vi "Default_Wash.vi"(0 "UI_Cluster_In":T1, 3 "error in":errorcluster) -> (7 "UI_Cluster_Out":T1, 10 "error out":errorcluster)   [LabVIEW 2020]
uses:
  controls/UI_Ref_Cluster.ctl
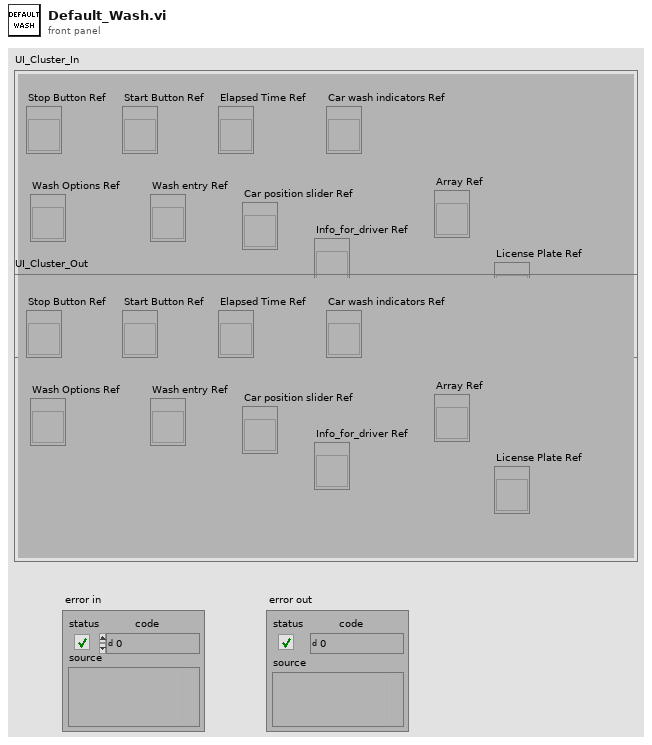
[diagram p1: front panel]
types:
  T1 = typedef "UI_Ref_Cluster.ctl" = cluster{"Stop Button Ref":refnum<vi>, "Start Button Ref":refnum<vi>, "Elapsed Time Ref":refnum<vi>, "Car wash indicators Ref":refnum<vi>, "Wash Options Ref":refnum<vi>, "Wash entry Ref":refnum<vi>, "Car position slider Ref":refnum<vi>, "Info_for_driver Ref":refnum<vi>, "Array Ref":refnum<vi>, "License Plate Ref":refnum<vi>}
  T2 = enum8{"Enabled", "Disabled", "Disabled and Grayed Out"}
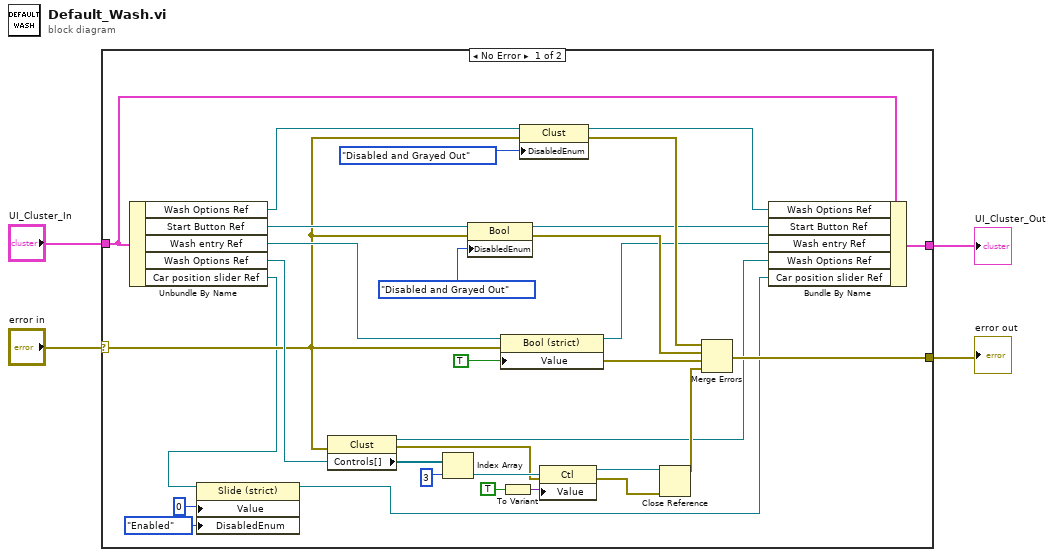
[diagram p0: block diagram]
diagram:
  n1 = case shown="No Error" "error in" {
    selector: "error in" -> [w15 w37]
    tunnel: [w21 w37] -> w3
    tunnel: "UI_Cluster_In" -> [w35 w36]
    tunnel: [w34 w36] -> w1
    frame No Error {
      n2 = Unbundle By Name(w35) -> ("Wash Options Ref"=w30:refnum<vi>, "Start Button Ref"=w27:refnum<vi>, "Wash entry Ref"=w24:refnum<vi>, "Wash Options Ref"=w20:refnum<vi>, "Car position slider Ref"=w7:refnum<vi>)
      n3 = property class="Slide (strict)"(reference=w7, "Value"=i8 0, "DisabledEnum"=T2."Enabled" ("Disabled")) -> (reference out=w6:refnum<vi>)  [unwired: 1 in, 1 out]
      n4 = property class="Clust"(reference=w20, error in=w15) -> (reference out=w9:refnum<vi>, error out=w14:errorcluster, "Controls[]"=w13:refnum<vi>[])
      n5 = Index Array(array=w13, index=3) -> (element=w18:refnum<vi>)
      n6 = property class="Bool"(reference=w27, error in=w15, "DisabledEnum"=T2."Disabled and Grayed Out" ("Disabled")) -> (reference out=w26:refnum<vi>, error out=w25:errorcluster)
      n7 = property class="Bool (strict)"(reference=w24, error in=w15, "Value"=TRUE) -> (reference out=w23:refnum<vi>, error out=w22:errorcluster)
      n8 = To Variant(anything=TRUE) -> (Variant=w16:variant)
      n9 = property class="Clust"(reference=w30, error in=w15, "DisabledEnum"=T2."Disabled and Grayed Out" ("Disabled")) -> (reference out=w28:refnum<vi>, error out=w29:errorcluster)
      n10 = property class="Ctl"(reference=w18, error in=w14, "Value"=w16) -> (reference out=w12:refnum<vi>, error out=w11:errorcluster)
      n11 = Close Reference(reference=w12, error in (no error)=w11) -> (error out=w10:errorcluster)
      n12 = Merge Errors(w29, w25, w22, w10) -> (w21:errorcluster)
      n13 = Bundle By Name(cluster=w35, "Wash Options Ref"=w28, "Start Button Ref"=w26, "Wash entry Ref"=w23, "Wash Options Ref"=w9, "Car position slider Ref"=w6) -> (w34:T1)
    }
    frame Error {
    }
  }
  "UI_Cluster_Out" <- w1
  "error out" <- w3
